vi "LWXPS_PositionerSGammaExactVelocityAjustedDisplacementGet.vi"(0 "XPS Reference IN":refnum<k24>, 5 "Positioner Name":string, 7 "Desired displacement":dbl, 11 "LabVIEW error IN":errorcluster) -> (4 "XPS Reference OUT":refnum<k24>, 6 "Returned error code":i32, 8 "Ajusted displacement":dbl, 10 "XPS Error String":string, 15 "LabVIEW error OUT":errorcluster)   [LabVIEW 2014]
uses:
  D:/XPSQ8_LabView_Library/Development/Source/Dll/Newport.XPS.CommandInterface.dll
  Dll/Newport.XPS.CommandInterface.dll
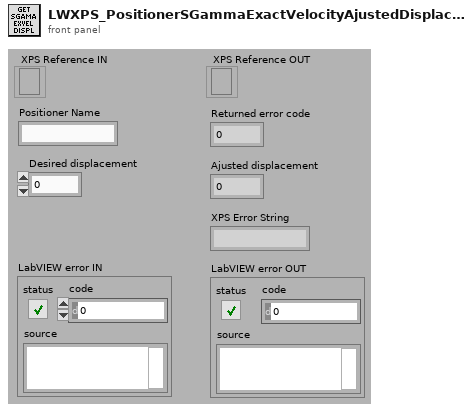
[diagram p1: front panel]
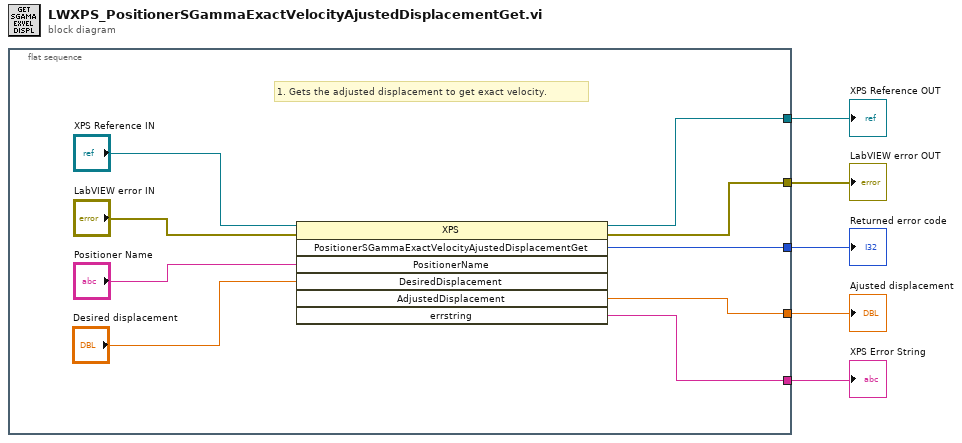
[diagram p0: block diagram]
diagram:
  n1 = flat-sequence {
    tunnel: [w12] -> w5
    tunnel: [w9] -> w4
    tunnel: [w13] -> w3
    tunnel: [w8] -> w2
    tunnel: [w7] -> w1
    frame #0 {
      # "1. Gets the adjusted displacement to get exact velocity."
      n2 = invoke class="XPS" method="PositionerSGammaExactVelocityAjustedDisplacementGet"(reference="XPS Reference IN", error in="LabVIEW error IN", "PositionerName"="Positioner Name", "DesiredDisplacement"="Desired displacement") -> (reference out=w12:refnum<k24>, error out=w9:errorcluster, "PositionerSGammaExactVelocityAjustedDisplacementGet"=w13:i32, "AdjustedDisplacement"=w8:dbl, "errstring"=w7:string)  [unwired: 3 in, 2 out]
    }
  }
  "XPS Error String" <- w1
  "XPS Reference OUT" <- w5
  "LabVIEW error OUT" <- w4
  "Returned error code" <- w3
  "Ajusted displacement" <- w2
